vi "command-processor.vi"(8 "error in":errorcluster, 10 "Variant":variant, 11 "Queue in":refnum<queue>) -> (0 "error out":errorcluster, 1 "Message Cluster 2":T1, 2 "delta 5":dbl, 3 "output cluster":T3)   [LabVIEW 2017]
uses:
  support/Message Queue/Message Cluster.ctl
  support/lib/event-message-data.ctl
  support/Message Queue/Enqueue Message (Single).vi
  support/Message Queue/Message Queue.lvlib
panel:
  in  "event-data":T2={"command-stack"=[""], "stack-config"=""}
  out "value 2":cluster{"address":i32}
  out "value":cluster{"command":string}
  out "command":string
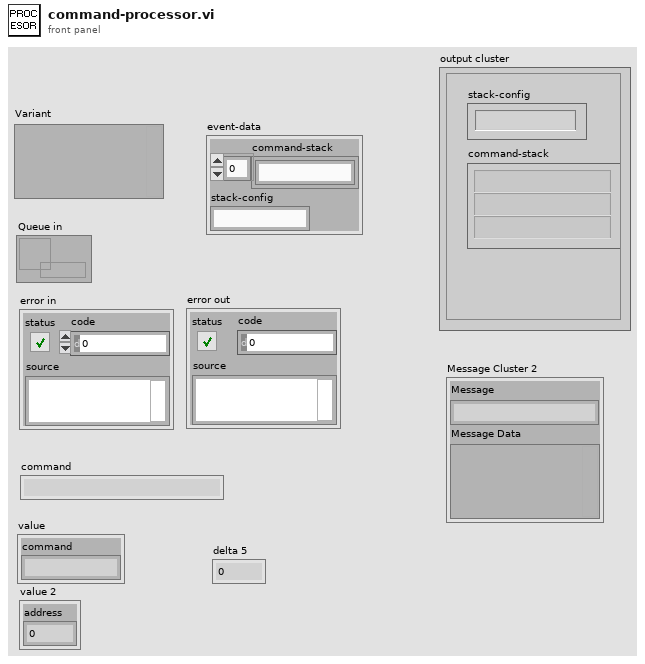
[diagram p1: front panel]
types:
  T1 = typedef "Message Queue.lvlib/Message Cluster.ctl" = cluster{"Message":string, "Message Data":variant}
  T2 = cluster{"command-stack":string[], "stack-config":string}
  T3 = typedef "event-message-data.ctl" = cluster{"command-stack":string[], "stack-config":string}
  T4 = cluster{"Label":string, "Instruction":string, "command":string, "address":i32}
  T5 = cluster{"_timestamp":dbl, "seconds":dbl, "inst":string}
  T6 = cluster{"label":string, "counter":u32, "_jumps":i64}
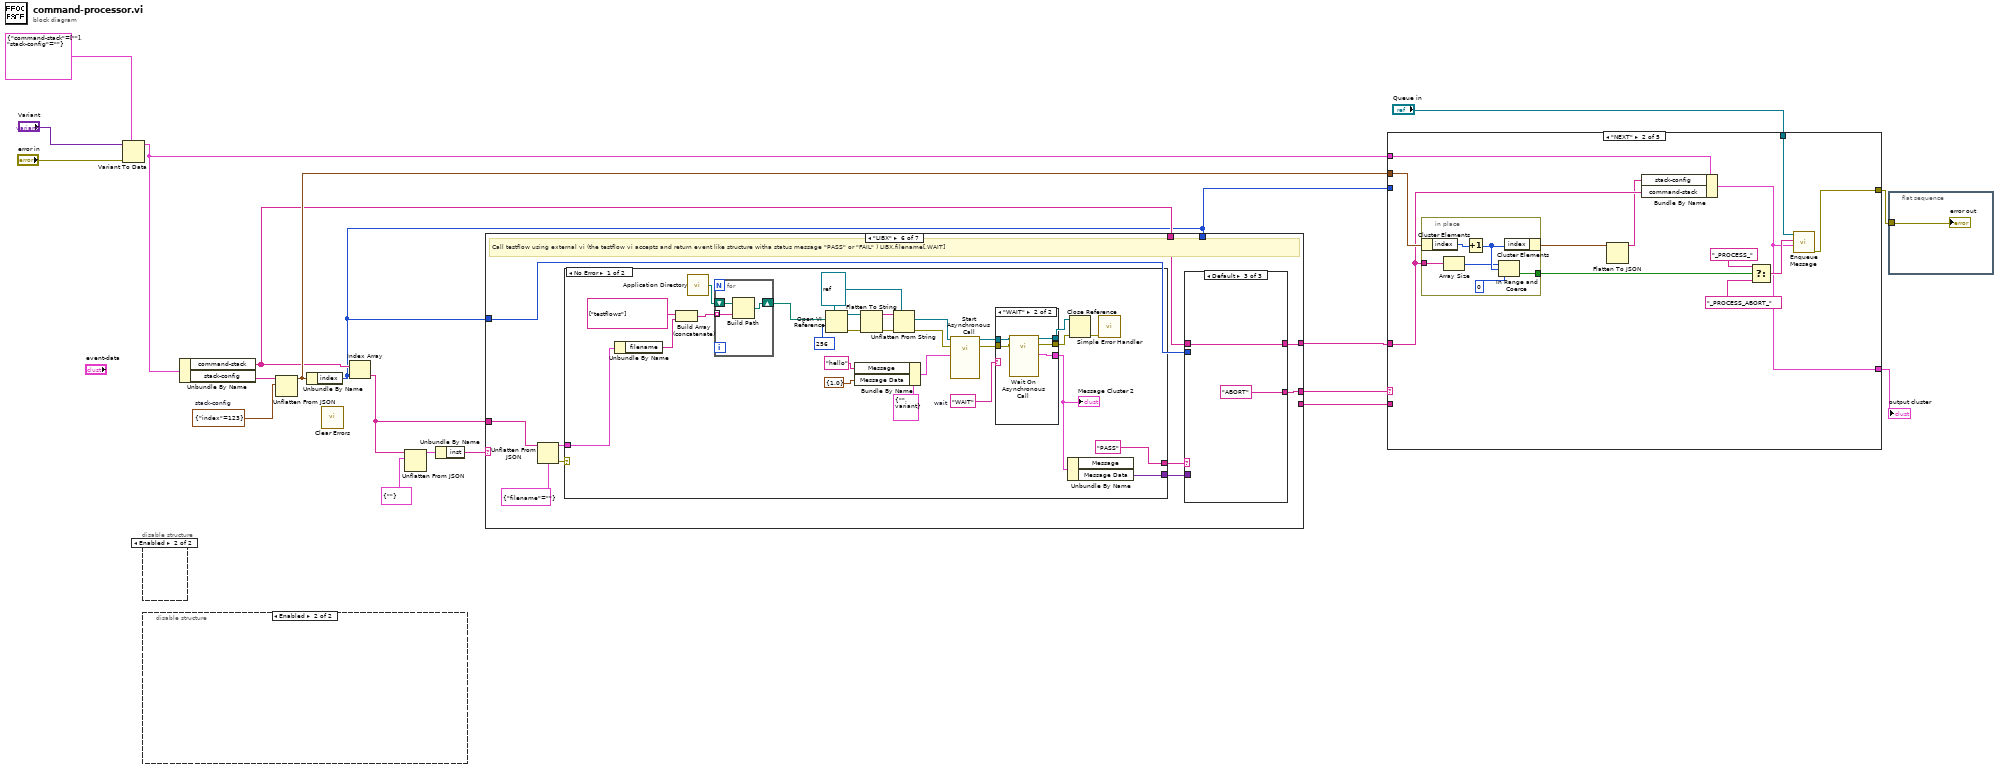
[diagram p0: block diagram]
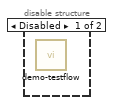
[diagram p2: hidden frame]
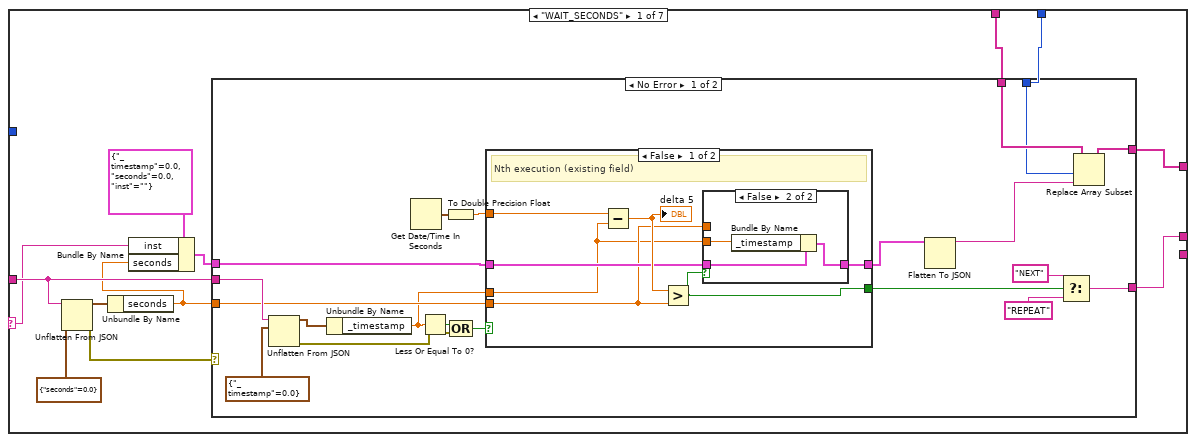
[diagram p3: hidden frame]
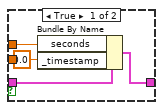
[diagram p4: hidden frame]
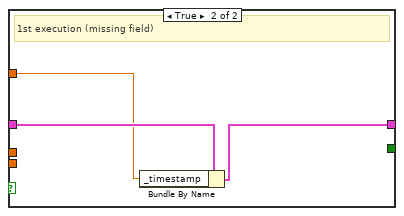
[diagram p5: hidden frame]
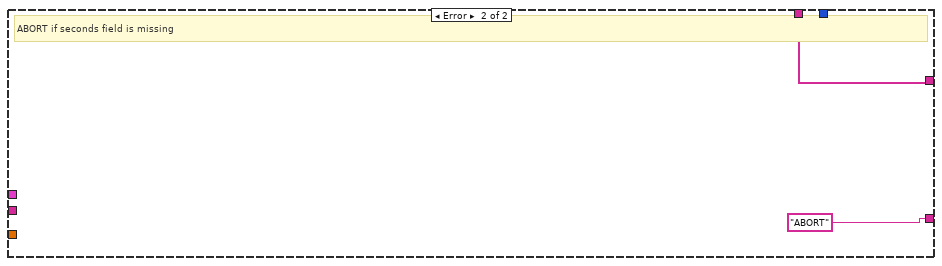
[diagram p6: hidden frame]
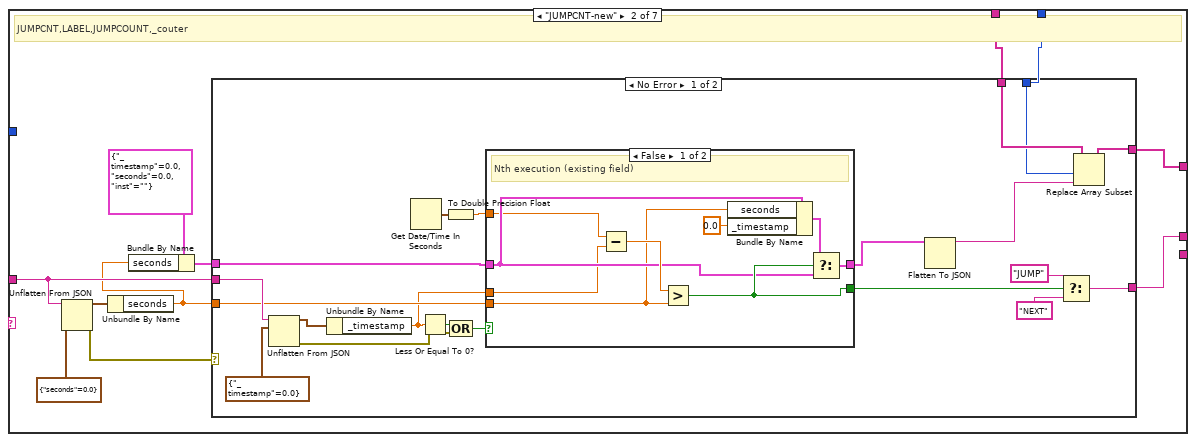
[diagram p7: hidden frame]
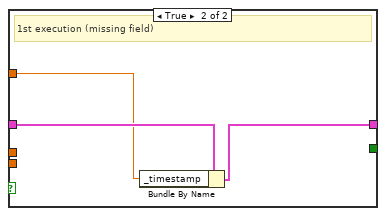
[diagram p8: hidden frame]
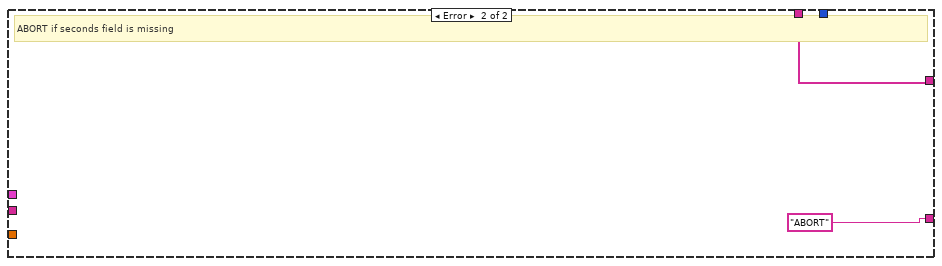
[diagram p9: hidden frame]
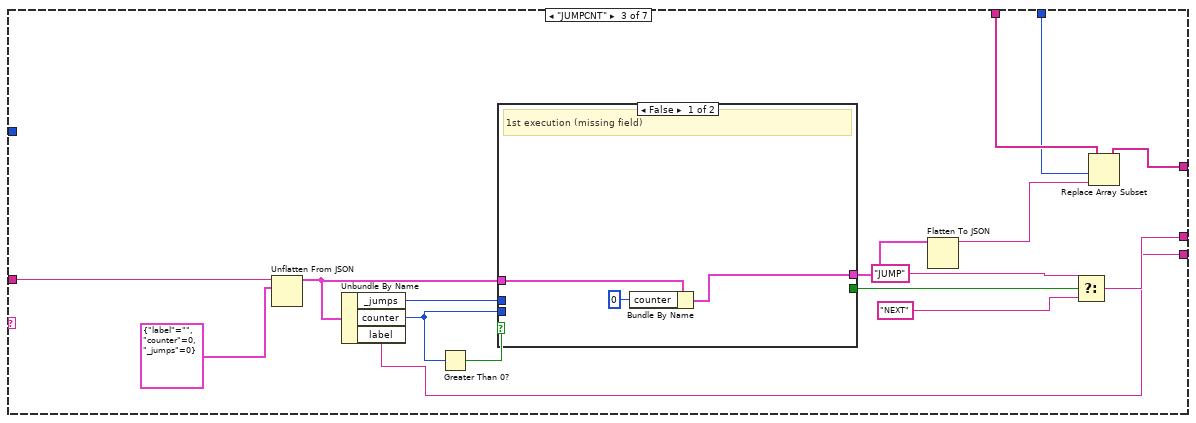
[diagram p10: hidden frame]
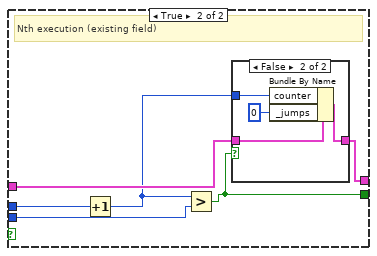
[diagram p11: hidden frame]
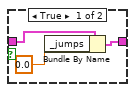
[diagram p12: hidden frame]
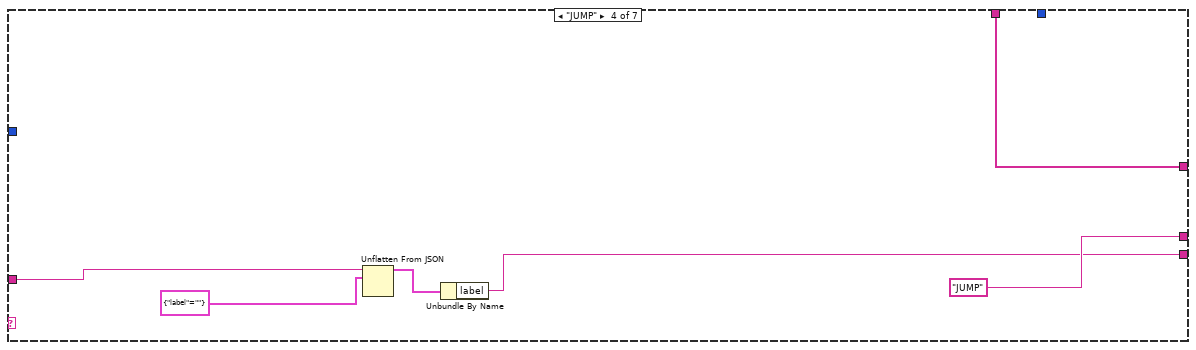
[diagram p13: hidden frame]
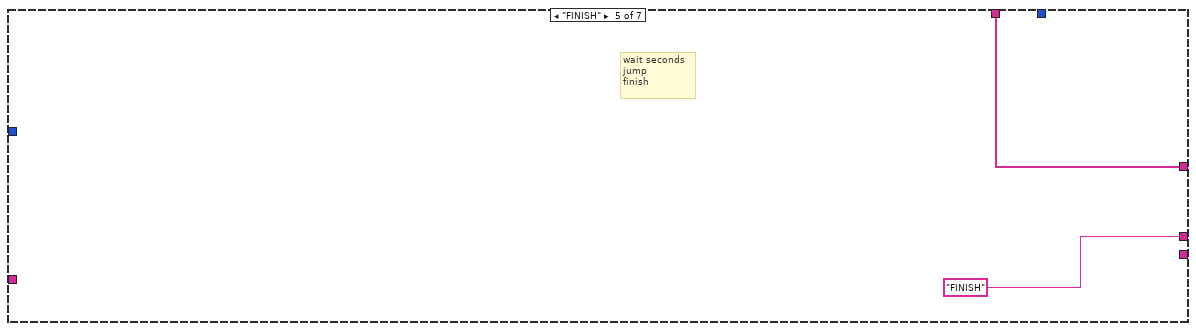
[diagram p14: hidden frame]
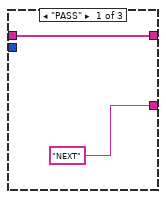
[diagram p17: hidden frame]
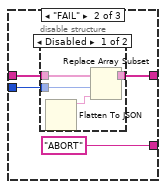
[diagram p18: hidden frame]
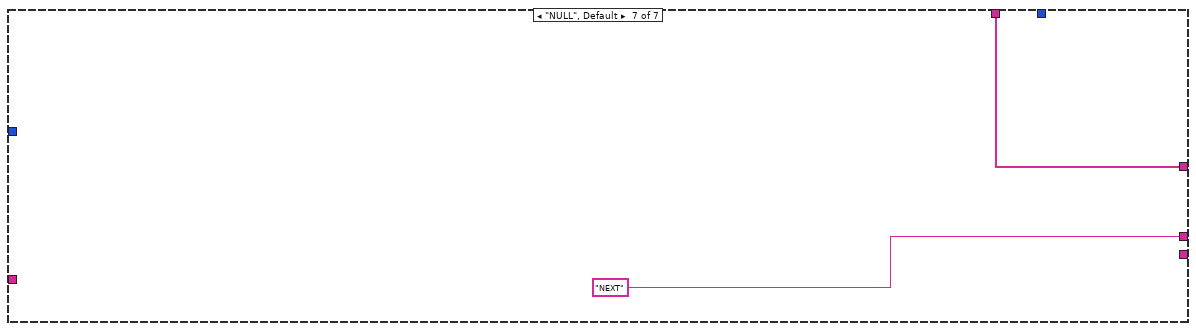
[diagram p20: hidden frame]
diagram:
  w6 = cluster{"index":i32} {"index"=123}  # stack-config
  n1 = Variant To Data(error in="error in", type=T3 {"command-stack"=[""], "stack-config"=""} ("process-unit"), Variant="Variant") -> (data=w4:T3)  [unwired: 1 out]
  n2 = disable-structure shown="Enabled" {
    frame Disabled {
      n3 = call "demo-testflow.vi"() -> ()  [unwired: 11 in, 1 out]
    }
    frame Enabled {
    }
  }
  n4 = disable-structure shown="Enabled" {
    frame Disabled {
      w21 = ""  # Label
      w20 = ""  # Instruction
      w26 = 123  # address
      w29 = "walla"  # command
      w22 = 123  # address
      w31 = "walla"  # command
      # "JSON command bus"
      n5 = Bundle("Label"=w21, "Instruction"=w20, "command"=w31, "address"=w22) -> (w30:T4)  [unwired: 1 in]
      n6 = Flatten To JSON(anything=w30) -> (JSON string=w25:string)  [unwired: 2 in, 1 out]
      "command" <- w25
      n7 = Bundle("command"=w29) -> (w28:cluster{"command":string})  [unwired: 1 in]
      n8 = Bundle("address"=w26) -> (w24:cluster{"address":i32})  [unwired: 1 in]
      n9 = Unflatten From JSON(JSON string=w25, type and defaults=w28) -> (value=→"value":cluster{"command":string})  [unwired: 5 in, 1 out]
      n10 = Unflatten From JSON(JSON string=w25, type and defaults=w24) -> (value=→"value 2":cluster{"address":i32})  [unwired: 5 in, 1 out]
    }
    frame Enabled {
    }
  }
  n11 = Unbundle By Name(w4) -> ("command-stack"=w3:string[], "stack-config"=w13:string)
  n12 = Unflatten From JSON(JSON string=w13, type and defaults=w6) -> (value=w5:cluster{"index":i32})  [unwired: 5 in, 1 out]
  n13 = Unbundle By Name(w5) -> ("index"=w2:i32)
  n14 = call <vilib>:"Clear Errors.vi"() -> ()  [unwired: 6 in, 2 out]
  n15 = Index Array(array=w3, index=w2) -> (element=w10:string)
  n16 = Unflatten From JSON(JSON string=w10, type and defaults=cluster{"inst":string} {"inst"=""} ("process-unit")) -> (value=w11:cluster{"inst":string})  [unwired: 5 in, 1 out]
  n17 = Unbundle By Name(w11) -> ("inst"=w9:string)
  n18 = case shown="\"LIBX\"" w9 {
    selector: w9 -> [w32 _ _ _ _ _ _]
    tunnel: [w43 w93 w142 "JUMP" ("format string") "FINISH" ("format string") w177 "NEXT" ("format string")] -> w8
    tunnel: [_ _ w128 w160 _ _ _] -> w7
    tunnel: w3 -> [w42 w92 w138 w164 w166 w170 w228]
    tunnel: w2 -> [w41 w91 w137 _ _ _ _]
    tunnel: [w40 w90 w136 w164 w166 w169 w228] -> w1
    tunnel: w10 -> [w39 w89 w134 w161 _ w174 _]
    tunnel: w2 -> [_ _ _ _ _ w171 _]
    frame "WAIT_SECONDS" {
      n19 = Unflatten From JSON(JSON string=w39, type and defaults=cluster{"seconds":dbl} {"seconds"=0.0} ("process-unit")) -> (value=w36:cluster{"seconds":dbl}, error out=w37:errorcluster)  [unwired: 5 in]
      n20 = Unbundle By Name(w36) -> ("seconds"=w33:dbl)
      n21 = Bundle By Name(cluster=T5 {"_timestamp"=0.0, "seconds"=0.0, "inst"=""} ("process-unit"), "inst"=w32, "seconds"=w33) -> (w34:T5)
      n22 = case shown="No Error" w37 {
        tunnel: [w63 "ABORT" ("format string")] -> w43
        tunnel: w42 -> [w59 w81]
        tunnel: w41 -> [w58 _]
        tunnel: [w57 w81] -> w40
        tunnel: w39 -> [w52 _]
        tunnel: w34 -> [w46 _]
        tunnel: w33 -> [w49 _]
        frame No Error {
          n23 = Unflatten From JSON(JSON string=w52, type and defaults=cluster{"_timestamp":dbl} {"_timestamp"=0.0} ("process-unit")) -> (value=w48:cluster{"_timestamp":dbl}, error out=w53:errorcluster)  [unwired: 5 in]
          n24 = Unbundle By Name(w48) -> ("_timestamp"=w47:dbl)
          n25 = Get Date/Time In Seconds() -> (seconds since 1Jan1904=w45:timestamp)
          n26 = Less Or Equal To 0?(x=w47) -> (x <= 0?=w50:bool)
          n27 = To Double Precision Float(number=w45) -> (double precision float=w44:dbl)
          n28 = Compound Arithmetic op=OR(w50, w53) -> (w51:bool)
          n29 = case shown="False" w51 {
            tunnel: [w65 _] -> w60
            tunnel: w46 -> [w69 w80]
            tunnel: [w68 w79] -> w55
            tunnel: w49 -> [w67 _]
            tunnel: w47 -> [w64 _]
            tunnel: w44 -> [w66 w78]
            frame False {
              # "Nth execution (existing field)"
              n30 = Subtract(x=w66, y=w64) -> (x-y=w70:dbl)
              "delta 5" <- w70
              n31 = Greater?(x=w70, y=w67) -> (0:w65:bool)
              n32 = case shown="False" w65 {
                tunnel: w69 -> [w74 w77]
                tunnel: [w71 w76] -> w68
                tunnel: w67 -> [w72 _]
                tunnel: w64 -> [_ w75]
                frame True {
                  n33 = Bundle By Name(cluster=w74, "seconds"=w72, "_timestamp"=0.0 ("seconds")) -> (w71:T5)
                }
                frame False {
                  n34 = Bundle By Name(cluster=w77, "_timestamp"=w75) -> (w76:T5)
                }
              }
            }
            frame True {
              # "1st execution (missing field)"
              n35 = Bundle By Name(cluster=w80, "_timestamp"=w78) -> (w79:T5)
            }
          }
          n36 = Flatten To JSON(anything=w55) -> (JSON string=w54:string)  [unwired: 2 in, 1 out]
          n37 = Select(t="NEXT" ("format string"), s=w60, f="REPEAT" ("format string")) -> (s? t:f=w63:string)
          n38 = Replace Array Subset(array=w59, new element=w54, index=w58) -> (w57:string[])
        }
        frame Error {
          # "ABORT if seconds field is missing"
        }
      }
    }
    frame "JUMPCNT-new" {
      # "JUMPCNT,LABEL,JUMPCOUNT,_couter"
      n39 = Unflatten From JSON(JSON string=w89, type and defaults=cluster{"seconds":dbl} {"seconds"=0.0} ("process-unit")) -> (value=w86:cluster{"seconds":dbl}, error out=w87:errorcluster)  [unwired: 5 in]
      n40 = Unbundle By Name(w86) -> ("seconds"=w83:dbl)
      n41 = Bundle By Name(cluster=T5 {"_timestamp"=0.0, "seconds"=0.0, "inst"=""} ("process-unit"), "seconds"=w83) -> (w84:T5)
      n42 = case shown="No Error" w87 {
        tunnel: [w113 "ABORT" ("format string")] -> w93
        tunnel: w92 -> [w109 w126]
        tunnel: w91 -> [w108 _]
        tunnel: [w107 w126] -> w90
        tunnel: w89 -> [w102 _]
        tunnel: w84 -> [w96 _]
        tunnel: w83 -> [w99 _]
        frame No Error {
          n43 = Unflatten From JSON(JSON string=w102, type and defaults=cluster{"_timestamp":dbl} {"_timestamp"=0.0} ("process-unit")) -> (value=w98:cluster{"_timestamp":dbl}, error out=w103:errorcluster)  [unwired: 5 in]
          n44 = Unbundle By Name(w98) -> ("_timestamp"=w97:dbl)
          n45 = Get Date/Time In Seconds() -> (seconds since 1Jan1904=w95:timestamp)
          n46 = Less Or Equal To 0?(x=w97) -> (x <= 0?=w100:bool)
          n47 = To Double Precision Float(number=w95) -> (double precision float=w94:dbl)
          n48 = Compound Arithmetic op=OR(w100, w103) -> (w101:bool)
          n49 = case shown="False" w101 {
            tunnel: [w121 _] -> w110
            tunnel: w96 -> [w120 w125]
            tunnel: [w119 w124] -> w105
            tunnel: w99 -> [w115 _]
            tunnel: w97 -> [w116 _]
            tunnel: w94 -> [w114 w123]
            frame False {
              # "Nth execution (existing field)"
              n50 = Subtract(x=w114, y=w116) -> (x-y=w122:dbl)
              n51 = Greater?(x=w122, y=w115) -> (0:w121:bool)
              n52 = Bundle By Name(cluster=w120, "seconds"=w115, "_timestamp"=0.0 ("seconds")) -> (w117:T5)
              n53 = Select(t=w117, s=w121, f=w120) -> (s? t:f=w119:T5)
            }
            frame True {
              # "1st execution (missing field)"
              n54 = Bundle By Name(cluster=w125, "_timestamp"=w123) -> (w124:T5)
            }
          }
          n55 = Flatten To JSON(anything=w105) -> (JSON string=w104:string)  [unwired: 2 in, 1 out]
          n56 = Select(t="JUMP" ("format string"), s=w110, f="NEXT" ("format string")) -> (s? t:f=w113:string)
          n57 = Replace Array Subset(array=w109, new element=w104, index=w108) -> (w107:string[])
        }
        frame Error {
          # "ABORT if seconds field is missing"
        }
      }
    }
    frame "JUMPCNT" {
      n58 = Unflatten From JSON(JSON string=w134, type and defaults=T6 {"label"="", "counter"=0, "_jumps"=0} ("process-unit")) -> (value=w133:T6)  [unwired: 5 in, 1 out]
      n59 = Unbundle By Name(w133) -> ("_jumps"=w131:i64, "counter"=w132:u32, "label"=w128:string)
      n60 = Greater Than 0?(x=w132) -> (x > 0?=w143:bool)
      n61 = case shown="False" w143 {
        tunnel: [_ w152] -> w139
        tunnel: w133 -> [w146 w150]
        tunnel: w132 -> [_ w148]
        tunnel: w131 -> [_ w151]
        tunnel: [w145 w149] -> w130
        frame False {
          # "1st execution (missing field)"
          n62 = Bundle By Name(cluster=w146, "counter"=u32 0) -> (w145:T6)
        }
        frame True {
          # "Nth execution (existing field)"
          n63 = Increment(x=w151) -> (x+1=w147:i64)
          n64 = Greater?(x=w147, y=w148) -> (0:w152:bool)
          n65 = case shown="False" w152 {
            tunnel: w150 -> [w155 w159]
            tunnel: [w154 w158] -> w149
            tunnel: w147 -> [_ w157]
            frame True {
              n66 = Bundle By Name(cluster=w155, "_jumps"=0.0 ("seconds")) -> (w154:T6)
            }
            frame False {
              n67 = Bundle By Name(cluster=w159, "counter"=w157, "_jumps"=i64 0) -> (w158:T6)
            }
          }
        }
      }
      n68 = Flatten To JSON(anything=w130) -> (JSON string=w129:string)  [unwired: 2 in, 1 out]
      n69 = Select(t="JUMP" ("format string"), s=w139, f="NEXT" ("format string")) -> (s? t:f=w142:string)
      n70 = Replace Array Subset(array=w138, new element=w129, index=w137) -> (w136:string[])
    }
    frame "JUMP" {
      n71 = Unflatten From JSON(JSON string=w161, type and defaults=cluster{"label":string} {"label"=""} ("process-unit")) -> (value=w162:cluster{"label":string})  [unwired: 5 in, 1 out]
      n72 = Unbundle By Name(w162) -> ("label"=w160:string)
    }
    frame "FINISH" {
      # "wait seconds \njump\nfinish"
    }
    frame "LIBX" {
      # "Call testflow using external vi (the testflow vi accepts and return event like structure witha status message \"PASS\" or \"FAIL\" ) LIBX,filename[,WAIT]"
      n73 = Unflatten From JSON(JSON string=w174, type and defaults=cluster{"filename":string} {"filename"=""} ("process-unit")) -> (value=w176:cluster{"filename":string}, error out=w168:errorcluster)  [unwired: 5 in]
      n74 = case shown="No Error" w168 {
        tunnel: w176 -> [w188 _]
        tunnel: ["PASS" ("Message") _] -> w173
        tunnel: [w179 _] -> w172
        frame No Error {
          w187 = "WAIT"  # wait
          w186 = refnum<vi> refnum ("type specifier VI Refnum (for type only)")
          n75 = Unbundle By Name(w188) -> ("filename"=w181:string)
          n76 = Build Array (concatenate)(string[] ["testflows"] ("name or relative path"), w181) -> (w182:string[])
          n77 = call <vilib>:"Application Directory.vi"() -> ("Application Directory"=w185:path)
          n78 = for {
            tunnel: w182 -> [w206] mode=indexing
            shift-right: [w205] -> w183
            shift-left: w185 -> [w207]
            n79 = Build Path(base path=w207, name or relative path=w206) -> (appended path=w205:path)
          }
          n80 = Open VI Reference(type specifier VI Refnum (for type only)=w186, vi path=w183, options=256 ("call and collect")) -> (vi reference=w195:refnum<vi>, error out=w193:errorcluster)  [unwired: 3 in]
          n81 = Bundle By Name(cluster=T1 {"Message"="", "Message Data"=variant} ("Message Cluster"), "Message"="hello", "Message Data"=cluster{"X":dbl} {"X"=1.0} ("output cluster")) -> (w204:T1)
          n82 = Flatten To String(anything=w195, error in (no error)=w193) -> (data string=w196:string, error out=w194:errorcluster)  [unwired: 2 in, 1 out]
          n83 = Unflatten From String(type=w186, binary string=w196, error in (no error)=w194) -> (value=w192:refnum<vi>, error out=w189:errorcluster)  [unwired: 2 in, 1 out]
          n84 = call-by-ref "Start Asynchronous Call"(reference=w192, error in=w189, "Message Cluster"=w204) -> (reference out=w191:refnum<vi>, error out=w190:errorcluster)  [unwired: 10 in, 1 out]
          n85 = case shown="\"WAIT\"" w187 {
            tunnel: [_ w214] -> w180
            tunnel: [w208 w213] -> w202
            tunnel: [w209 w212] -> w201
            tunnel: w191 -> [w209 w211]
            tunnel: w190 -> [w208 w210]
            frame Default {
            }
            frame "WAIT" {
              n86 = call-by-ref "Wait On Asynchronous Call"(reference=w211, error in=w210) -> (reference out=w212:refnum<vi>, error out=w213:errorcluster, "Message Cluster 2"=w214:T1)  [unwired: 11 in]
            }
          }
          "Message Cluster 2" <- w180
          n87 = Unbundle By Name(w180) -> ("Message Data"=w179:variant)  [unwired: 1 out]
          n88 = Close Reference(reference=w201, error in (no error)=w202) -> (error out=w200:errorcluster)
          n89 = call <vilib>:"Simple Error Handler.vi"("error in (no error)"=w200) -> ()  [unwired: 4 in, 5 out]
        }
        frame Error {
        }
      }
      n90 = case shown="Default" w173 {
        tunnel: ["NEXT" ("format string") "ABORT" ("format string") "ABORT" ("format string")] -> w177
        tunnel: w172 -> [_ _ _]
        tunnel: w170 -> [w215 w219 w226]
        tunnel: w171 -> [_ w218 _]
        tunnel: [w215 w217 w226] -> w169
        frame "PASS" {
        }
        frame "FAIL" {
          n91 = disable-structure shown="Disabled" {
            disable-tunnel: w219 -> [w223 w225]
            disable-tunnel: w218 -> [w222 _]
            disable-tunnel: [w221 w225] -> w217
            frame Disabled {
              n92 = Flatten To JSON() -> (JSON string=w224:string)  [unwired: 3 in, 1 out]
              n93 = Replace Array Subset(array=w223, new element=w224, index=w222) -> (w221:string[])
            }
            frame Enabled {
            }
          }
        }
        frame Default {
        }
      }
    }
    frame "NULL", Default {
    }
  }
  n94 = case shown="\"NEXT\"" w8 {
    tunnel: "Queue in" -> [w234 w248 w263 w270 w285]
    tunnel: [w233 w247 w262 w269 w284] -> w14
    tunnel: w7 -> [_ _ _ _ w282]
    tunnel: w2 -> [_ _ _ _ _]
    tunnel: [w231 w242 w260 w267 w283] -> w16
    tunnel: w4 -> [w232 w243 w261 w266 w277]
    tunnel: w1 -> [w230 w240 w258 w265 w276]
    tunnel: w5 -> [_ w241 w259 _ w272]
    frame "REPEAT" {
      n95 = Bundle By Name(cluster=w232, "command-stack"=w230) -> (w231:T3)
      n96 = To Variant(anything=w231) -> (Variant=w235:variant)
      n97 = call-poly "Enqueue Message.vi"("Message Data"=w235, "Message"="_PROCESS_", "Message Queue"=w234) -> ("error out"=w233:errorcluster)  [unwired: 7 in, 1 out]
    }
    frame "NEXT" {
      n98 = in-place {
        in-place-border: w240 -> [w250]
        in-place-border: [w249] -> w239
        n99 = in-place-cluster #1(w241) -> ("index"=w254:i32)
        n100 = Array Size(array=w250) -> (size(s)=w251:i32)
        n101 = Increment(x=w254) -> (x+1=w252:i32)
        n102 = In Range and Coerce(upper limit=w251, x=w252, lower limit=i64 0) -> (In Range?=w249:bool)  [unwired: 1 out]
        n103 = in-place-cluster #1("index"=w252) -> (w237:cluster{"index":i32})
      }
      n104 = Flatten To JSON(anything=w237) -> (JSON string=w238:string)  [unwired: 2 in, 1 out]
      n105 = Bundle By Name(cluster=w243, "stack-config"=w238, "command-stack"=w240) -> (w242:T3)
      n106 = Select(t="_PROCESS_" ("Message"), s=w239, f="_PROCESS_ABORT_" ("Message")) -> (s? t:f=w244:string)
      n107 = call-poly "Enqueue Message.vi"("Message Data"=w242, "Message"=w244, "Message Queue"=w248) -> ("error out"=w247:errorcluster)  [unwired: 7 in, 1 out]
    }
    frame "ABORT", Default {
      n108 = in-place {
        in-place-border: w258 -> [_]
        n109 = in-place-cluster #2(w259) -> ("index"=w264:i32)
        n110 = in-place-cluster #2("index"=w264) -> (w257:cluster{"index":i32})
      }
      n111 = Flatten To JSON(anything=w257) -> (JSON string=w256:string)  [unwired: 2 in, 1 out]
      n112 = Bundle By Name(cluster=w261, "stack-config"=w256, "command-stack"=w258) -> (w260:T3)
      n113 = call-poly "Enqueue Message.vi"("Message Data"=w260, "Message"="_PROCESS_ABORT_", "Message Queue"=w263) -> ("error out"=w262:errorcluster)  [unwired: 7 in, 1 out]
    }
    frame "FINISH" {
      n114 = Bundle By Name(cluster=w266, "command-stack"=w265) -> (w267:T3)
      n115 = To Variant(anything=w267) -> (Variant=w271:variant)
      n116 = call-poly "Enqueue Message.vi"("Message Data"=w271, "Message"="_PROCESS_FINISH_", "Message Queue"=w270) -> ("error out"=w269:errorcluster)  [unwired: 7 in, 1 out]
    }
    frame "JUMP" {
      n117 = for "SEARCH INSTRUCTION BY LABEL" {
        tunnel: w276 -> [w291] mode=indexing
        tunnel: [w295] -> w274
        tunnel: w282 -> [w288]
        tunnel: [w293] -> w280
        i -> [w295]
        stop <- w293 stop-if-true
        n118 = Unflatten From JSON(JSON string=w291, type and defaults=cluster{"label":string} {"label"=""} ("process-unit")) -> (value=w290:cluster{"label":string})  [unwired: 5 in, 1 out]
        n119 = Unbundle(w290) -> ("label"=w289:string)
        n120 = Equal?(x=w288, y=w289) -> (x = y?=w294:bool)
        n121 = Compound Arithmetic op=AND(w294) -> (w293:bool)
      }
      n122 = in-place {
        in-place-border: w274 -> [w287]
        n123 = in-place-cluster #3(w272) -> ()  [unwired: 1 out]
        n124 = in-place-cluster #3("index"=w287) -> (w275:cluster{"index":i32})
      }
      n125 = Select(t="_PROCESS_" ("Message"), s=w280, f="_PROCESS_ERROR_JUMP" ("Message")) -> (s? t:f=w278:string)
      n126 = Flatten To JSON(anything=w275) -> (JSON string=w273:string)  [unwired: 2 in, 1 out]
      n127 = Bundle By Name(cluster=w277, "stack-config"=w273, "command-stack"=w276) -> (w283:T3)
      n128 = To Variant(anything=w283) -> (Variant=w286:variant)
      n129 = call-poly "Enqueue Message.vi"("Message Data"=w286, "Message"=w278, "Message Queue"=w285) -> ("error out"=w284:errorcluster)  [unwired: 7 in, 1 out]
    }
  }
  "output cluster" <- w16
  n130 = flat-sequence {
    tunnel: w14 -> [w296]
    frame #0 {
      "error out" <- w296
    }
  }
